vi "Install and Uninstall Components.vi"(6 "Install Options":T1={"version selection (highest)"=[], "auto-select dependencies (T)"=TRUE, "auto-select recommended (F)"=FALSE} {"version selection (highest)" items=["Highest", "Exactly"]}, 7 "Restart Automatically (T)":bool=TRUE, 8 "error in (no error)":errorcluster, 9 "Software IDs to Uninstall":string[](array[string]), 10 "Software Components to Install":T3[](array[typedef]) {"component type" items=["standard", "hidden", "system", "unknown", "startup", "image", "essential"]}, 11 "Session in":refnum<k21>) -> (0 "error out":errorcluster, 1 "Broken Dependencies":T2[](array[typedef]) {"dependee"."component type" items=["standard", "hidden", "system", "unknown", "startup", "image", "essential"]; "depender"."component type" items=["standard", "hidden", "system", "unknown", "startup", "image", "essential"]}, 3 "Session out":refnum<k21>)   [LabVIEW 2017, in "nisyscfg.lvlib"]
doc: "Use the Install and Uninstall Components VI to install components, uninstall components, or both install and uninstall components simultaneously (as long as two components do not overlap each other).\n\nThis VI installs components you specify in the <B>Software Components to Install</B> parameter, as well as any required hidden components. If <B>Auto-select Dependencies</B> is TRUE, this VI also installs other visible components if they are dependencies of any component you specified to install in the <B>Software Components to Install</B> parameter and they are not already installed on the system. This VI only uninstalls visible components that are specified in the <B>Software IDs to Uninstall</B> parameter."
uses:
  <vilib>/nisyscfg/nisyscfg.lvlib
  <vilib>/nisyscfg/Software 1.2.ctl
  <vilib>/nisyscfg/Component Type.ctl
  <vilib>/nisyscfg/Broken Dependency 1.2.ctl
  <vilib>/nisyscfg/Install Options.ctl
  <vilib>/Utility/error.llb/Error Cluster From Error Code.vi
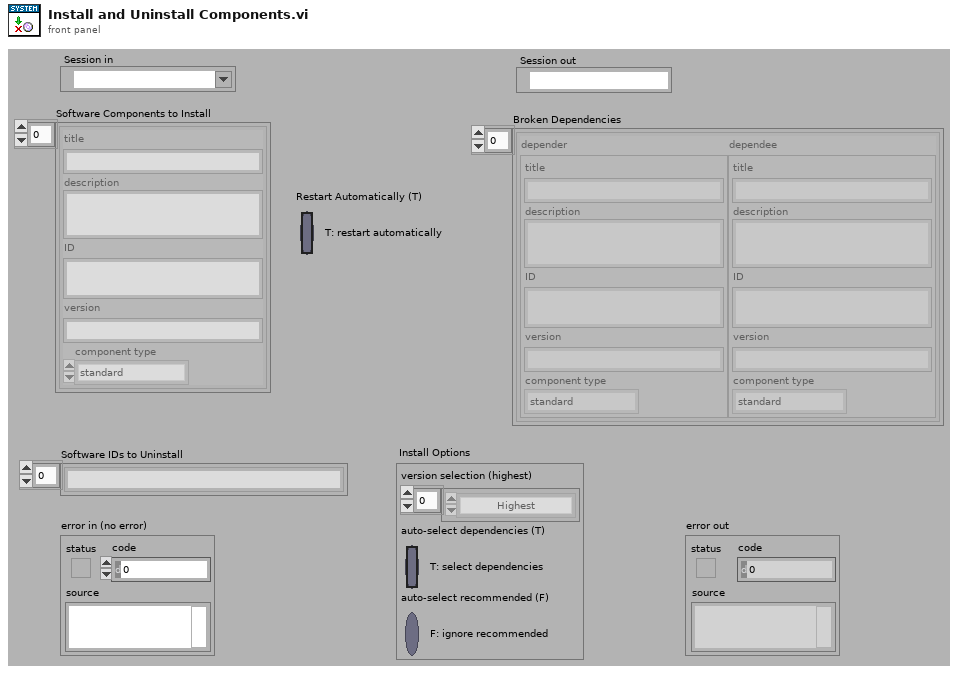
[diagram p1: front panel]
types:
  T1 = typedef "nisyscfg.lvlib/Install Options.ctl" = cluster{"version selection (highest)":u32[], "auto-select dependencies (T)":bool, "auto-select recommended (F)":bool}
  T2 = typedef "nisyscfg.lvlib/Broken Dependency 1.2.ctl" = cluster{"depender":T3, "dependee":T3}
  T3 = typedef "nisyscfg.lvlib/Software 1.2.ctl" = cluster{"title":string, "description":string, "ID":string, "version":string, "component type":T4}
  T4 = typedef "nisyscfg.lvlib/Component Type.ctl" = u32
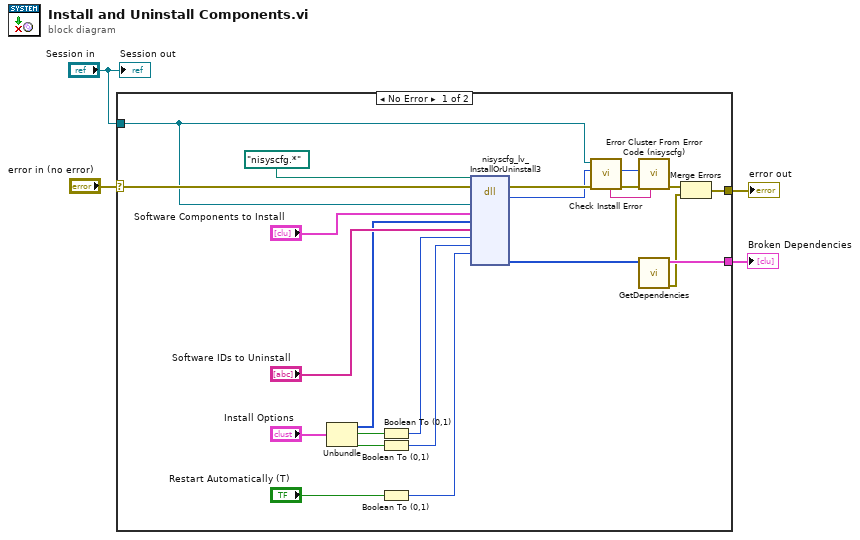
[diagram p0: block diagram]
diagram:
  n1 = case shown="No Error" "error in (no error)" {
    selector: "error in (no error)" -> [w17 w28]
    tunnel: "Session in" -> [w16 _]
    tunnel: [w18 w28] -> w4
    tunnel: [w23 _] -> w3
    frame No Error {
      n2 = Unbundle("Install Options") -> ("version selection (highest)"=w7:u32[], "auto-select dependencies (T)"=w6:bool, "auto-select recommended (F)"=w5:bool)
      n3 = Boolean To (0,1)(Boolean=w6) -> (0, 1=w25:i16)
      n4 = Boolean To (0,1)(Boolean=w5) -> (0, 1=w9:i16)
      n5 = Boolean To (0,1)(Boolean="Restart Automatically (T)") -> (0, 1=w19:i16)
      n6 = dll-call lib="nisyscfg.*" fn="nisyscfg_lv_InstallOrUninstall3" label="InstallOrUninstall3"(path in=path "nisyscfg.*", error in=w17, "session"=w16, "softwareToInstall"="Software Components to Install", "versionSelectionMode"=w7, "softwareIDsToUninstall"="Software IDs to Uninstall", "autoSelectDependencies"=w25, "autoSelectRecommends"=w9, "restartAutomatically"=w19) -> (error out=w15:errorcluster, "result"=w14:i32, "brokenDependencies"=w24:u64[])  [unwired: 9 in, 1 out]
      n7 = call <vilib>:"Check Install Error.vi"("error in (no error)"=w15, "Status in"=w14, "Session in"=w16) -> ("error out"=w12:errorcluster, "Status out"=w13:i32, "Details"=w10:string)  [unwired: 5 in, 1 out]
      n8 = call <vilib>:"Error Cluster From Error Code (nisyscfg).vi"("Details String"=w10, "error in (no error)"=w12, "Error Code (0)"=w13) -> ("error out"=w11:errorcluster)  [unwired: 8 in]
      n9 = call <vilib>:"GetDependencies.vi"("Enumerator in"=w24) -> ("error out"=w21:errorcluster, "Dependencies"=w23:T2[])  [unwired: 9 in]
      n10 = Merge Errors(w11, w21) -> (w18:errorcluster)
    }
    frame Error {
    }
  }
  "error out" <- w4
  "Broken Dependencies" <- w3
  "Session out" <- "Session in"
